vi "Main.vi"() -> ()   [LabVIEW 2015]
doc: "This small application is only a proof of concept. When we have parameters or user data inside an application that could be modified (by the user) at run time, it is important that those changes are 'memorized' when the application is shut down. The next time the application is started it should keep the last configuration made. This is what this application does.\n\nEvery time the user changes the FP data, the changes are saved in the .ini file. If the user closes the application, the FP data is already saved in the .ini configuration file. The next time it is turned on, the data will be loaded again.\n\nIf the user modifies any tag or sector name, or any key name (or its value) in the configuration file (and saves these changes) at run time, the Update button updates this information in the FP of the application, it is the data of the gray fields. This may not be useful in a real application."
uses:
  support/Message Queue/Message Queue.lvlib
  <vilib>/Utility/error.llb/Error Cluster From Error Code.vi
  support/User Event - Stop/User Event - Stop.lvlib
  support/Message Queue/Enqueue Message (Single).vi
  <vilib>/ErrorRing/Error Ring.xnode
  support/Message Queue/Enqueue Message (Array).vi
  controls/UI Data.ctl
  controls/user data.ctl
panel:
  in  "Update":bool
  out "Sector3":string
  out "Sector2":string
  out "Sector1":string
  out "key22":string
  out "key21":string
  out "key13":string
  out "key12":string
  out "key11":string
  in  "value32":string
  out "key32":string
  in  "value31":string
  out "key31":string
  in  "value22":string
  in  "value13":string
  in  "value21":string
  in  "value12":string
  in  "value11":string
  out "Display value":string
  in  "Exit":bool
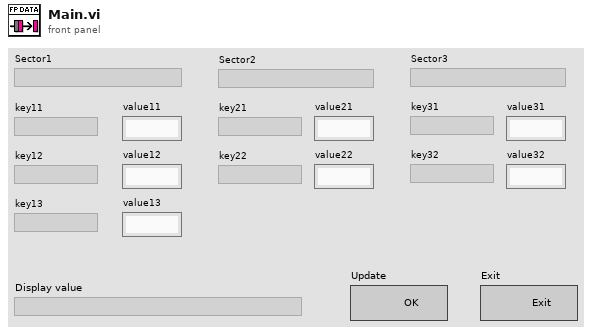
[diagram p1: front panel]
types:
  T1 = typedef "UI Data.ctl" = cluster{"Data Display Ref":refnum<vi>, "Exit Button Ref":refnum<vi>, "Update Ref":refnum<vi>, "sector ref":refnum<vi>[], "key ref":refnum<vi>[][], "value ref":refnum<vi>[][], "user data":T2}
  T2 = typedef "user data.ctl" = cluster{"sector":string[][], "key names":string[][], "values":string[][]}
  T3 = typedef "Message Queue.lvlib/All Message Queues.ctl" = cluster{"UI":refnum<queue>}
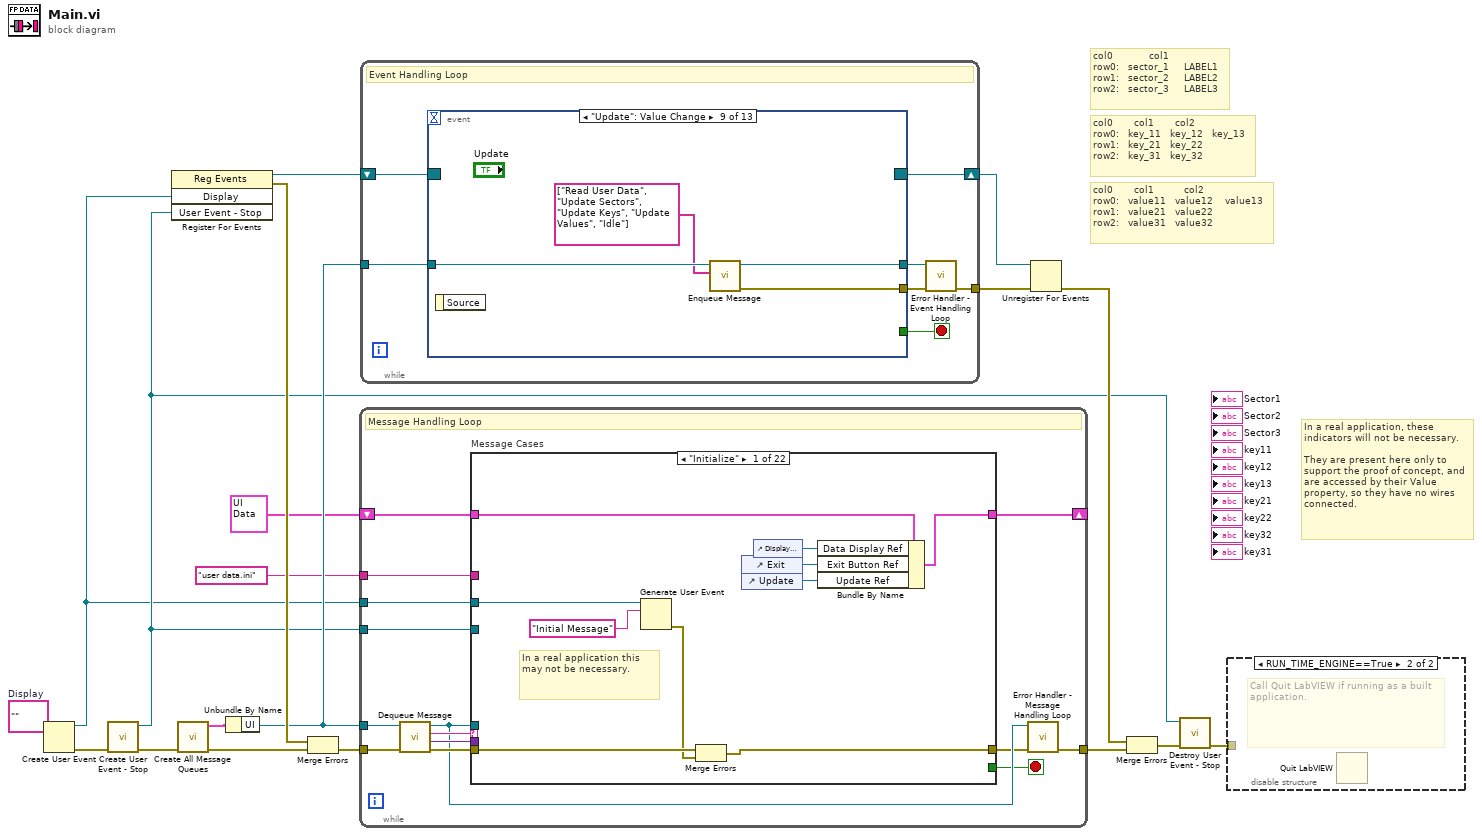
[diagram p0: block diagram]
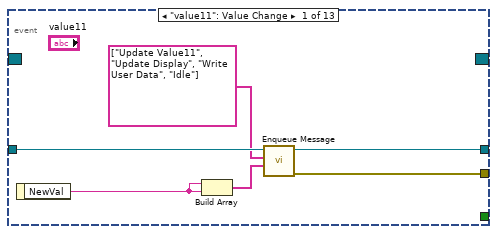
[diagram p3: hidden frame]
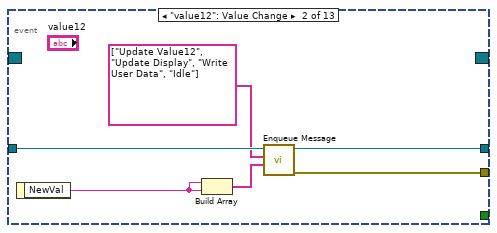
[diagram p4: hidden frame]
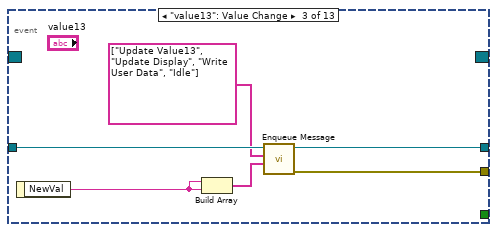
[diagram p5: hidden frame]
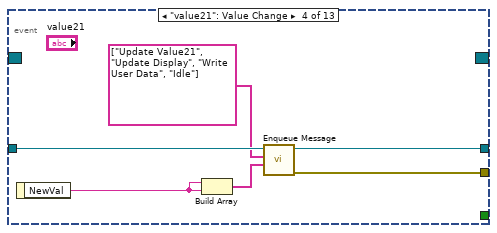
[diagram p6: hidden frame]
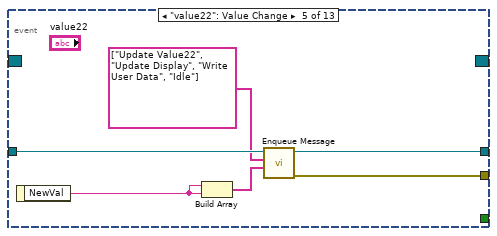
[diagram p7: hidden frame]
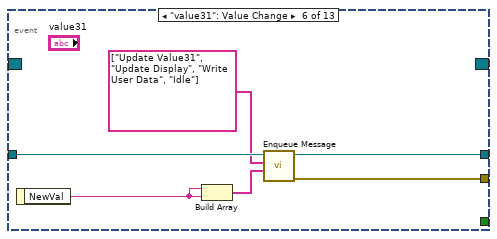
[diagram p8: hidden frame]
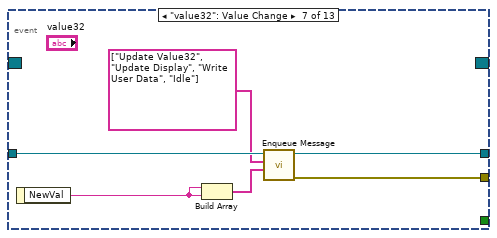
[diagram p9: hidden frame]
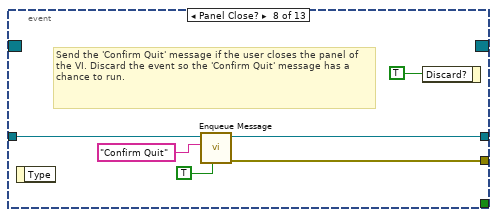
[diagram p10: hidden frame]
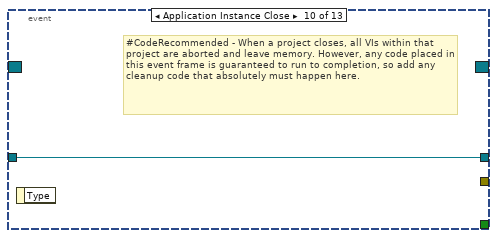
[diagram p11: hidden frame]
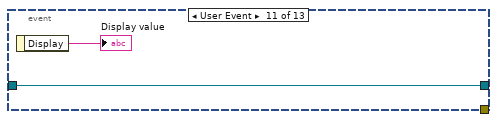
[diagram p12: hidden frame]
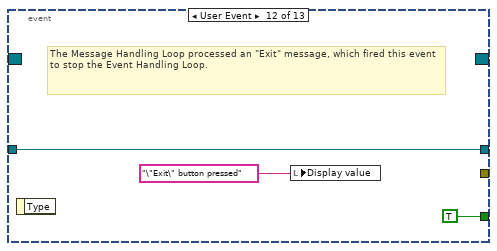
[diagram p13: hidden frame]
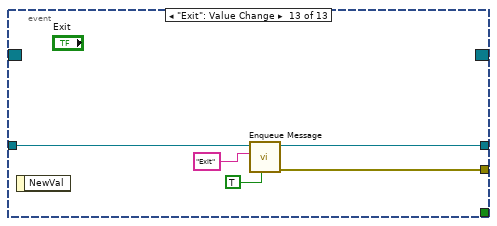
[diagram p14: hidden frame]
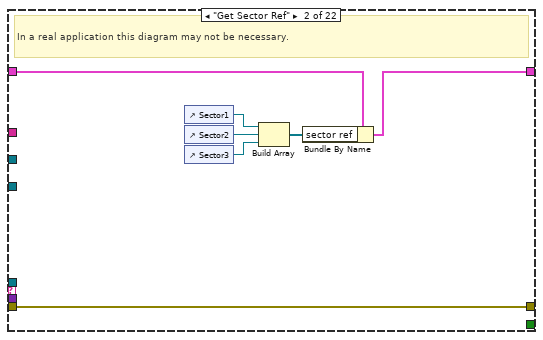
[diagram p15: hidden frame]
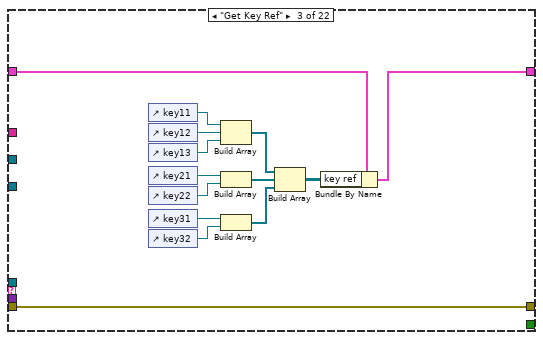
[diagram p16: hidden frame]
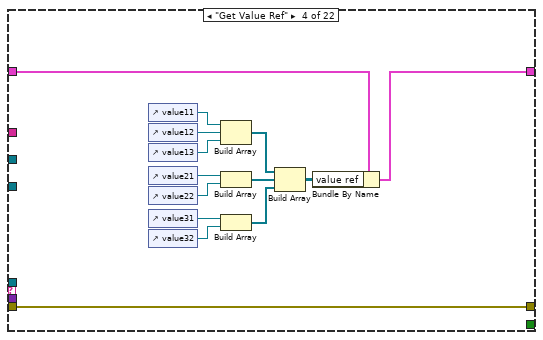
[diagram p17: hidden frame]
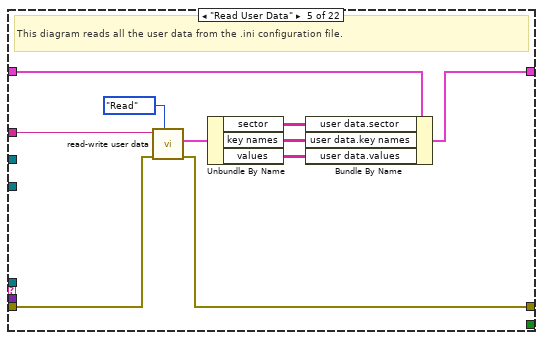
[diagram p18: hidden frame]
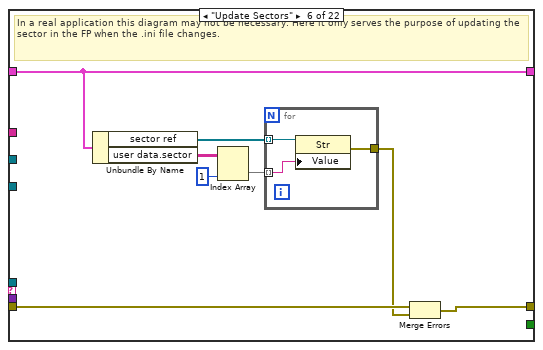
[diagram p19: hidden frame]
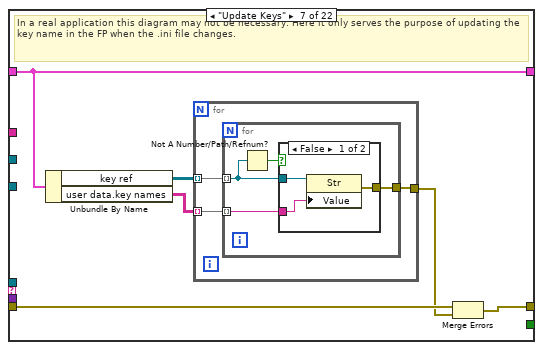
[diagram p20: hidden frame]
diagram:
  w4 = ""  # Display
  # "In a real application, these indicators will not be necessary. \n\nThey are present here only to support the proof of concept, and are accessed by their Value property, so they have no wires connected."
  # "col0       col1          col2\nrow0:   value11   value12    value13\nrow1:   value21   value22\nrow2:   value31   value32"
  # "col0       col1       col2\nrow0:   key_11   key_12   key_13\nrow1:   key_21   key_22 \nrow2:   key_31   key_32"
  # "col0            col1\nrow0:   sector_1     LABEL1\nrow1:   sector_2     LABEL2\nrow2:   sector_3     LABEL3"
  n1 = Create User Event(user event datatype=w4) -> (user event=w2:refnum<user-event>, error out=w5:errorcluster)  [unwired: 1 in]
  n2 = call "Create User Event - Stop.vi"("error in (no error)"=w5) -> ("error out"=w14:errorcluster, "User Event - Stop"=w3:refnum<user-event>)  [unwired: 9 in]
  n3 = register-events(w2, w3) -> (reference out=w7:refnum<event-registration>, error out=w19:errorcluster)  [unwired: 2 in]
  n4 = call "Create All Message Queues.vi"("error in (no error)"=w14) -> ("error out"=w18:errorcluster, "Message Queues out"=w17:T3)  [unwired: 9 in]
  n5 = Unbundle By Name(w17) -> ("UI"=w15:refnum<queue>)
  n6 = Merge Errors(w19, w18) -> (w6:errorcluster)
  n7 = while {
    tunnel: w15 -> [w27]
    shift-right: [w22] -> _
    shift-left: T1 {"Data Display Ref"=refnum, "Exit Button Ref"=refnum, "Update Ref"=refnum, "sector ref"=[], "key ref"=[], "value ref"=[], "user data"={"sector"=[], "key names"=[], "values"=[]}} ("Data Cluster") -> [w33]
    tunnel: w3 -> [w32]
    tunnel: w6 -> [w31]
    tunnel: [w25] -> w16
    tunnel: w2 -> [w23]
    tunnel: "user data.ini" -> [w21]
    stop <- w20 stop-if-true
    # "Message Handling Loop"
    n8 = call "Dequeue Message.vi"("error in (no error)"=w31, "Message Queue"=w27) -> ("error out"=w30:errorcluster, "Message Data"=w28:variant, "Message"=w29:string, "dup Message Queue"=w26:refnum<queue>)  [unwired: 6 in]
    n9 = case "Message Cases" shown="\"Initialize\"" w29 {
      selector: w29 -> [_ _ _ _ _ _ _ _ _ _ _ _ _ _ _ _ _ _ _ _ _ w252]
      tunnel: w26 -> [_ _ _ _ _ _ _ _ _ _ _ _ _ _ _ _ _ _ w233 _ w251 _]
      tunnel: w30 -> [w39 w50 w64 w78 w85 w96 w105 w121 w141 w152 w163 w174 w185 w196 w207 w210 w221 w230 w237 w240 w244 _]
      tunnel: [w36 w50 w64 w78 w84 w90 w103 w119 w140 w151 w162 w173 w184 w195 w206 w209 w222 w224 w235 w238 w247 w253] -> w24
      tunnel: w33 -> [w43 w49 w63 w77 w88 w95 w104 w120 w137 w148 w159 w170 w181 w192 w203 w214 w223 w229 w236 w239 w250 w254]
      tunnel: [w42 w48 w62 w76 w87 w95 w104 w120 w142 w153 w164 w175 w186 w197 w208 w214 w223 w229 w236 w239 w250 w254] -> w22
      tunnel: [_ _ _ _ _ _ _ _ _ _ _ _ _ _ _ _ _ _ _ _ TRUE _] -> w20
      tunnel: w28 -> [_ _ _ _ _ _ _ _ w138 w149 w160 w171 w182 w193 w204 _ w220 w228 _ _ w241 _]
      tunnel: w32 -> [_ _ _ _ _ _ _ _ _ _ _ _ _ _ _ _ _ _ _ _ w246 _]
      tunnel: w23 -> [w38 _ _ _ _ _ _ _ _ _ _ _ _ _ _ _ w217 _ _ _ _ _]
      tunnel: w21 -> [_ _ _ _ w79 _ _ _ _ _ _ _ _ _ _ w211 _ _ _ _ _ _]
      frame "Initialize" {
        # "In a real application this may not be necessary."
        n10 = Generate User Event(user event=w38, event data cluster="Initial Message" ("Initial Message")) -> (error out=w35:errorcluster)  [unwired: 2 in, 1 out]
        n11 = Merge Errors(w39, w35) -> (w36:errorcluster)
        n12 = control-ref of="Exit"() -> (w40:refnum<vi>)
        n13 = control-ref of="Update"() -> (w34:refnum<vi>)
        n14 = control-ref of="Display value"() -> (w41:refnum<vi>)
        n15 = Bundle By Name(cluster=w43, "Data Display Ref"=w41, "Exit Button Ref"=w40, "Update Ref"=w34) -> (w42:T1)
      }
      frame "Get Sector Ref" {
        # "In a real application this diagram may not be necessary."
        n16 = control-ref of="Sector1"() -> (w47:refnum<vi>)
        n17 = control-ref of="Sector2"() -> (w45:refnum<vi>)
        n18 = control-ref of="Sector3"() -> (w46:refnum<vi>)
        n19 = Build Array(w47, w45, w46) -> (w44:refnum<vi>[])
        n20 = Bundle By Name(cluster=w49, "sector ref"=w44) -> (w48:T1)
      }
      frame "Get Key Ref" {
        n21 = control-ref of="key11"() -> (w61:refnum<vi>)
        n22 = control-ref of="key12"() -> (w59:refnum<vi>)
        n23 = control-ref of="key13"() -> (w60:refnum<vi>)
        n24 = control-ref of="key21"() -> (w57:refnum<vi>)
        n25 = control-ref of="key22"() -> (w58:refnum<vi>)
        n26 = control-ref of="key31"() -> (w56:refnum<vi>)
        n27 = control-ref of="key32"() -> (w55:refnum<vi>)
        n28 = Build Array(w61, w59, w60) -> (w54:refnum<vi>[])
        n29 = Build Array(w57, w58) -> (w53:refnum<vi>[])
        n30 = Build Array(w56, w55) -> (w52:refnum<vi>[])
        n31 = Build Array(w54, w53, w52) -> (w51:refnum<vi>[][])
        n32 = Bundle By Name(cluster=w63, "key ref"=w51) -> (w62:T1)
      }
      frame "Get Value Ref" {
        n33 = control-ref of="value11"() -> (w75:refnum<vi>)
        n34 = control-ref of="value12"() -> (w73:refnum<vi>)
        n35 = control-ref of="value13"() -> (w74:refnum<vi>)
        n36 = control-ref of="value21"() -> (w71:refnum<vi>)
        n37 = control-ref of="value22"() -> (w72:refnum<vi>)
        n38 = control-ref of="value31"() -> (w70:refnum<vi>)
        n39 = control-ref of="value32"() -> (w69:refnum<vi>)
        n40 = Build Array(w75, w73, w74) -> (w68:refnum<vi>[])
        n41 = Build Array(w71, w72) -> (w67:refnum<vi>[])
        n42 = Build Array(w70, w69) -> (w66:refnum<vi>[])
        n43 = Build Array(w68, w67, w66) -> (w65:refnum<vi>[][])
        n44 = Bundle By Name(cluster=w77, "value ref"=w65) -> (w76:T1)
      }
      frame "Read User Data" {
        # "This diagram reads all the user data from the .ini configuration file."
        n45 = call "read-write user data.vi"("Function"=enum16{"Read", "Write"}."Read", "error in (no error)"=w85, "file name"=w79) -> ("error out"=w84:errorcluster, "user data out"=w83:T2)  [unwired: 7 in]
        n46 = Unbundle By Name(w83) -> ("sector"=w82:string[][], "key names"=w81:string[][], "values"=w80:string[][])
        n47 = Bundle By Name(cluster=w88, "user data.sector"=w82, "user data.key names"=w81, "user data.values"=w80) -> (w87:T1)
      }
      frame "Update Sectors" {
        # "In a real application this diagram may not be necessary. Here it only serves the purpose of updating the sector in the FP when the .ini file changes."
        n48 = Unbundle By Name(w95) -> ("sector ref"=w94:refnum<vi>[], "user data.sector"=w93:string[][])
        n49 = Index Array(array=w93, index (col)=1 ("disabled index (col)")) -> (element=w91:string[])  [unwired: 1 in]
        n50 = for {
          tunnel: w94 -> [w99] mode=indexing
          tunnel: w91 -> [w98] mode=indexing
          tunnel: [w97] -> w89
          n51 = property class="Str"(reference=w99, "Value"=w98) -> (error out=w97:errorcluster)  [unwired: 1 in, 1 out]
        }
        n52 = Merge Errors(w96, w89) -> (w90:errorcluster)
      }
      frame "Update Keys" {
        # "In a real application this diagram may not be necessary. Here it only serves the purpose of updating the key name in the FP when the .ini file changes."
        n53 = Unbundle By Name(w104) -> ("key ref"=w101:refnum<vi>[][], "user data.key names"=w100:string[][])
        n54 = for {
          tunnel: w100 -> [w108] mode=indexing
          tunnel: [w107] -> w102
          tunnel: w101 -> [w106] mode=indexing
          n55 = for {
            tunnel: w108 -> [w112] mode=indexing
            tunnel: [w111] -> w107
            tunnel: w106 -> [w110] mode=indexing
            n56 = Not A Number/Path/Refnum?(number/path/refnum=w110) -> (NaN/Path/Refnum?=w109:bool)
            n57 = case shown="False" w109 {
              tunnel: w112 -> [w115 _]
              tunnel: [w114 _] -> w111
              tunnel: w110 -> [w113 _]
              frame False {
                n58 = property class="Str"(reference=w113, "Value"=w115) -> (error out=w114:errorcluster)  [unwired: 1 in, 1 out]
              }
              frame True {
              }
            }
          }
        }
        n59 = Merge Errors(w105, w102) -> (w103:errorcluster)
      }
      frame "Update Values" {
        # "This diagram is only executed when the application is started or the Update button is pressed. \nIt is used to update the value of the keys in the FP."
        n60 = Unbundle By Name(w120) -> ("value ref"=w117:refnum<vi>[][], "user data.values"=w116:string[][])
        n61 = for {
          tunnel: w116 -> [w124] mode=indexing
          tunnel: [w123] -> w118
          tunnel: w117 -> [w122] mode=indexing
          n62 = for {
            tunnel: w124 -> [w128] mode=indexing
            tunnel: [w127] -> w123
            tunnel: w122 -> [w126] mode=indexing
            n63 = Not A Number/Path/Refnum?(number/path/refnum=w126) -> (NaN/Path/Refnum?=w125:bool)
            n64 = case shown="False" w125 {
              tunnel: w128 -> [w131 _]
              tunnel: [w130 _] -> w127
              tunnel: w126 -> [w129 _]
              frame False {
                n65 = property class="Str"(reference=w129, "Value"=w131) -> (error out=w130:errorcluster)  [unwired: 1 in, 1 out]
              }
              frame True {
              }
            }
          }
        }
        n66 = Merge Errors(w121, w118) -> (w119:errorcluster)
      }
      frame "Update Value11" {
        n67 = Unbundle By Name(w137) -> ("user data.values"=w136:string[][])
        n68 = Variant To Data(error in=w141, type="", Variant=w138) -> (data=w134:string, error out=w140:errorcluster)
        n69 = Replace Array Subset(array=w136, new element=w134, index (row)=0, index (col)=0) -> (w135:string[][])
        n70 = Bundle By Name(cluster=w137, "user data.values"=w135) -> (w142:T1)
      }
      frame "Update Value12" {
        n71 = Unbundle By Name(w148) -> ("user data.values"=w147:string[][])
        n72 = Variant To Data(error in=w152, type="", Variant=w149) -> (data=w145:string, error out=w151:errorcluster)
        n73 = Replace Array Subset(array=w147, new element=w145, index (row)=0, index (col)=1) -> (w146:string[][])
        n74 = Bundle By Name(cluster=w148, "user data.values"=w146) -> (w153:T1)
      }
      frame "Update Value13" {
        n75 = Unbundle By Name(w159) -> ("user data.values"=w158:string[][])
        n76 = Variant To Data(error in=w163, type="", Variant=w160) -> (data=w156:string, error out=w162:errorcluster)
        n77 = Replace Array Subset(array=w158, new element=w156, index (row)=0, index (col)=2) -> (w157:string[][])
        n78 = Bundle By Name(cluster=w159, "user data.values"=w157) -> (w164:T1)
      }
      frame "Update Value21" {
        n79 = Unbundle By Name(w170) -> ("user data.values"=w169:string[][])
        n80 = Variant To Data(error in=w174, type="", Variant=w171) -> (data=w167:string, error out=w173:errorcluster)
        n81 = Replace Array Subset(array=w169, new element=w167, index (row)=1, index (col)=0) -> (w168:string[][])
        n82 = Bundle By Name(cluster=w170, "user data.values"=w168) -> (w175:T1)
      }
      frame "Update Value22" {
        n83 = Unbundle By Name(w181) -> ("user data.values"=w180:string[][])
        n84 = Variant To Data(error in=w185, type="", Variant=w182) -> (data=w178:string, error out=w184:errorcluster)
        n85 = Replace Array Subset(array=w180, new element=w178, index (row)=1, index (col)=1) -> (w179:string[][])
        n86 = Bundle By Name(cluster=w181, "user data.values"=w179) -> (w186:T1)
      }
      frame "Update Value31" {
        n87 = Unbundle By Name(w192) -> ("user data.values"=w191:string[][])
        n88 = Variant To Data(error in=w196, type="", Variant=w193) -> (data=w189:string, error out=w195:errorcluster)
        n89 = Replace Array Subset(array=w191, new element=w189, index (row)=2, index (col)=0) -> (w190:string[][])
        n90 = Bundle By Name(cluster=w192, "user data.values"=w190) -> (w197:T1)
      }
      frame "Update Value32" {
        n91 = Unbundle By Name(w203) -> ("user data.values"=w202:string[][])
        n92 = Variant To Data(error in=w207, type="", Variant=w204) -> (data=w200:string, error out=w206:errorcluster)
        n93 = Replace Array Subset(array=w202, new element=w200, index (row)=2, index (col)=1) -> (w201:string[][])
        n94 = Bundle By Name(cluster=w203, "user data.values"=w201) -> (w208:T1)
      }
      frame "Write User Data" {
        # "In this diagram all user data is written to the .ini configuration file."
        n95 = Unbundle By Name(w214) -> ("user data"=w212:T2)
        n96 = call "read-write user data.vi"("Function"=enum16{"Read", "Write"}."Write", "error in (no error)"=w210, "user data in"=w212, "file name"=w211) -> ("error out"=w209:errorcluster)  [unwired: 6 in, 1 out]
      }
      frame "Update Display" {
        # "In a real application this may not be necessary."
        # "Update Display - Convert the message data to a string to display in the Data Display indicator."
        n97 = Variant To Data(error in=w221, type="", Variant=w220) -> (data=w216:string, error out=w218:errorcluster)
        n98 = Generate User Event(user event=w217, event data cluster=w216) -> (error out=w215:errorcluster)  [unwired: 2 in, 1 out]
        n99 = Merge Errors(w218, w215) -> (w222:errorcluster)
      }
      frame "Error" {
        # "#CodeRecommended - If you ever change the name of this \"Error\" message, you'll need to update the name in the Check Loop Error.vi as well."
        # "#CodeRecommended - Consider creating a system for logging errors in some way. These errors are for notification purposes only. Handling of specific errors should be performed in the message frames that generated the error."
        # "Error - Display an error dialog. This message is sent by the \"Error Handler\" VIs at the end of other loops in this application."
        n100 = Variant To Data(error in=w230, type=errorcluster {"status"=FALSE, "code"=0, "source"=""} ("error constant"), Variant=w228) -> (data=w226:errorcluster, error out=w225:errorcluster)
        n101 = call <vilib>:"Simple Error Handler.vi"("error in (no error)"=w226) -> ()  [unwired: 4 in, 5 out]
        n102 = Merge Errors(w225) -> (w224:errorcluster)
      }
      frame "Confirm Quit" {
        # "#CodeNeeded - If you want to provide an \"Are you sure\" dialog (or some other notification) before the application exits, place that code here. This message is typically sent from a Panel Close? event."
        # "Confirm Quit - Message that can confirm whether or not the user wants to exit the application."
        n103 = call-poly "Enqueue Message.vi"("Priority Message? (F)"=TRUE, "error in (no error)"=w237, "Message"="Exit", "Message Queue"=w233) -> ("error out"=w234:errorcluster)  [unwired: 6 in, 1 out]
        n104 = Merge Errors(w234) -> (w235:errorcluster)
      }
      frame "Idle" {
        # "Idle diagram"
        n105 = Merge Errors(w240) -> (w238:errorcluster)
      }
      frame "Exit" {
        # "Release the message queue reference"
        # "#CodeNeeded - Add any required cleanup code here. Note that if 'Exit' was called as a result of an error, an error dialog will be displayed. Add any custom error handling for an 'Exit' condition here as well."
        # "Exit - Exit the application."
        n106 = Variant To Data(type=errorcluster {"status"=FALSE, "code"=0, "source"=""} ("error constant"), Variant=w241) -> (data=w242:errorcluster)  [unwired: 1 in, 1 out]
        n107 = call <vilib>:"Simple Error Handler.vi"("error in (no error)"=w242) -> ()  [unwired: 4 in, 5 out]
        n108 = call "Fire User Event - Stop.vi"("User Event - Stop"=w246) -> ("error out"=w245:errorcluster)  [unwired: 10 in]
        n109 = Release Queue(queue=w251, error in (no error)=w244) -> (error out=w248:errorcluster)  [unwired: 1 in, 2 out]
        n110 = Merge Errors(w245, w248) -> (w247:errorcluster)
      }
      frame Default {
        # "'Default' case only runs if there is a message that isn't defined in any of the other cases.  Output a programming error."
        n111 = xnode "Error Ring"("parameter 0"=w252) -> ("error out"=w253:errorcluster)
      }
    }
    n112 = call "Error Handler - Message Handling Loop.vi"("error in (no error)"=w24, "Message Queue"=w26) -> ("dup error in"=w25:errorcluster)  [unwired: 8 in, 1 out]
  }
  n113 = while {
    tunnel: w15 -> [w268]
    shift-right: [w266] -> w11
    shift-left: w7 -> [w267]
    tunnel: [w262] -> w8
    stop <- w264 stop-if-true
    # "Event Handling Loop"
    n114 = event shown="[8] \"Update\": Value Change" {
      selector: w267 -> [_ _ _ _ _ _ _ _ _ _ _ _ _]
      dyn-events: [_ _ _ _ _ _ _ _ _ _ _ _ _] -> w266
      timeout: _ -> [_ _ _ _ _ _ _ _ _ _ _ _ _]
      tunnel: [_ _ _ _ _ _ _ _ _ _ _ TRUE ("Discard?") _] -> w264
      tunnel: w268 -> [w274 w280 w286 w292 w298 w304 w310 w315 w320 w321 w323 w326 w331]
      tunnel: [w272 w278 w284 w290 w296 w302 w308 w314 w318 _ _ _ w330] -> w265
      tunnel: [w273 w279 w285 w291 w297 w303 w309 w313 w319 w321 w323 w326 w329] -> w263
      event "value11": Value Change {
        n115 = event-data() -> ("NewVal"=w269:string)  [unwired: 1 in]
        n116 = Build Array(w269, w269) -> (w270:string[])
        n117 = call-poly "Enqueue Message.vi"("Message Data Array"=w270, "Message Array"=string[] ["Update Value11", "Update Display", "Write User Data", "Idle"], "Message Queue"=w274) -> ("error out"=w272:errorcluster, "dup Message Queue"=w273:refnum<queue>)  [unwired: 7 in]
      }
      event "value12": Value Change {
        n118 = event-data() -> ("NewVal"=w275:string)  [unwired: 1 in]
        n119 = Build Array(w275, w275) -> (w276:string[])
        n120 = call-poly "Enqueue Message.vi"("Message Data Array"=w276, "Message Array"=string[] ["Update Value12", "Update Display", "Write User Data", "Idle"], "Message Queue"=w280) -> ("error out"=w278:errorcluster, "dup Message Queue"=w279:refnum<queue>)  [unwired: 7 in]
      }
      event "value13": Value Change {
        n121 = event-data() -> ("NewVal"=w281:string)  [unwired: 1 in]
        n122 = Build Array(w281, w281) -> (w282:string[])
        n123 = call-poly "Enqueue Message.vi"("Message Data Array"=w282, "Message Array"=string[] ["Update Value13", "Update Display", "Write User Data", "Idle"], "Message Queue"=w286) -> ("error out"=w284:errorcluster, "dup Message Queue"=w285:refnum<queue>)  [unwired: 7 in]
      }
      event "value21": Value Change {
        n124 = event-data() -> ("NewVal"=w287:string)  [unwired: 1 in]
        n125 = Build Array(w287, w287) -> (w288:string[])
        n126 = call-poly "Enqueue Message.vi"("Message Data Array"=w288, "Message Array"=string[] ["Update Value21", "Update Display", "Write User Data", "Idle"], "Message Queue"=w292) -> ("error out"=w290:errorcluster, "dup Message Queue"=w291:refnum<queue>)  [unwired: 7 in]
      }
      event "value22": Value Change {
        n127 = event-data() -> ("NewVal"=w293:string)  [unwired: 1 in]
        n128 = Build Array(w293, w293) -> (w294:string[])
        n129 = call-poly "Enqueue Message.vi"("Message Data Array"=w294, "Message Array"=string[] ["Update Value22", "Update Display", "Write User Data", "Idle"], "Message Queue"=w298) -> ("error out"=w296:errorcluster, "dup Message Queue"=w297:refnum<queue>)  [unwired: 7 in]
      }
      event "value31": Value Change {
        n130 = event-data() -> ("NewVal"=w299:string)  [unwired: 1 in]
        n131 = Build Array(w299, w299) -> (w300:string[])
        n132 = call-poly "Enqueue Message.vi"("Message Data Array"=w300, "Message Array"=string[] ["Update Value31", "Update Display", "Write User Data", "Idle"], "Message Queue"=w304) -> ("error out"=w302:errorcluster, "dup Message Queue"=w303:refnum<queue>)  [unwired: 7 in]
      }
      event "value32": Value Change {
        n133 = event-data() -> ("NewVal"=w305:string)  [unwired: 1 in]
        n134 = Build Array(w305, w305) -> (w306:string[])
        n135 = call-poly "Enqueue Message.vi"("Message Data Array"=w306, "Message Array"=string[] ["Update Value32", "Update Display", "Write User Data", "Idle"], "Message Queue"=w310) -> ("error out"=w308:errorcluster, "dup Message Queue"=w309:refnum<queue>)  [unwired: 7 in]
      }
      event Panel Close? {
        # "Send the 'Confirm Quit' message if the user closes the panel of the VI. Discard the event so the 'Confirm Quit' message has a chance to run."
        n136 = event-data() -> ()  [unwired: 1 in, 1 out]
        n137 = call-poly "Enqueue Message.vi"("Priority Message? (F)"=TRUE, "Message"="Confirm Quit", "Message Queue"=w315) -> ("error out"=w314:errorcluster, "dup Message Queue"=w313:refnum<queue>)  [unwired: 7 in]
        n138 = event-data("Discard?"=TRUE) -> ()  [unwired: 1 in, 1 out]
      }
      event "Update": Value Change {
        n139 = event-data() -> ()  [unwired: 1 in, 1 out]
        n140 = call-poly "Enqueue Message.vi"("Message Array"=string[] ["Read User Data", "Update Sectors", "Update Keys", "Update Values", "Idle"], "Message Queue"=w320) -> ("error out"=w318:errorcluster, "dup Message Queue"=w319:refnum<queue>)  [unwired: 8 in]
      }
      event Application Instance Close {
        # "#CodeRecommended - When a project closes, all VIs within that project are aborted and leave memory. However, any code placed in this event frame is guaranteed to run to completion, so add any cleanup code that absolutely must happen here."
        n141 = event-data() -> ()  [unwired: 1 in, 1 out]
      }
      event User Event {
        n142 = event-data() -> ("Display"=→"Display value":string)  [unwired: 1 in]
      }
      event User Event {
        # "The Message Handling Loop processed an \"Exit\" message, which fired this event to stop the Event Handling Loop."
        n143 = event-data() -> ()  [unwired: 1 in, 1 out]
        n144 = local write "Display value"("\"Exit\" button pressed" ("VI Stopped")) -> ()
      }
      event "Exit": Value Change {
        n145 = event-data() -> ()  [unwired: 1 in, 1 out]
        n146 = call-poly "Enqueue Message.vi"("Priority Message? (F)"=TRUE, "Message"="Exit", "Message Queue"=w331) -> ("error out"=w330:errorcluster, "dup Message Queue"=w329:refnum<queue>)  [unwired: 7 in]
      }
    }
    n147 = call "Error Handler - Event Handling Loop.vi"("error in (no error)"=w265, "Message Queue"=w263) -> ("dup error in"=w262:errorcluster)  [unwired: 8 in, 1 out]
  }
  n148 = Unregister For Events(event registration refnum=w11, error in=w8) -> (error out=w12:errorcluster)
  n149 = Merge Errors(w12, w16) -> (w13:errorcluster)
  n150 = call "Destroy User Event - Stop.vi"("error in (no error)"=w13, "User Event - Stop"=w3) -> ("error out"=w9:errorcluster)  [unwired: 9 in]
  n151 = disable-structure shown="RUN_TIME_ENGINE==True" {
    disable-tunnel: w9 -> [_ _]
    frame condition #0 (active) {
    }
    frame condition #1 {
      # "Call Quit LabVIEW if running as a built application."
      n152 = Quit LabVIEW() -> ()  [unwired: 1 in]
    }
  }
